vi "Data from tests for IGOR.vi"() -> ()   [LabVIEW 2020]
panel:
  out "G4T vs t Vacuum":cluster{dbl[], dbl[]}(graph)
  out "G4T vs t":T1(graph)
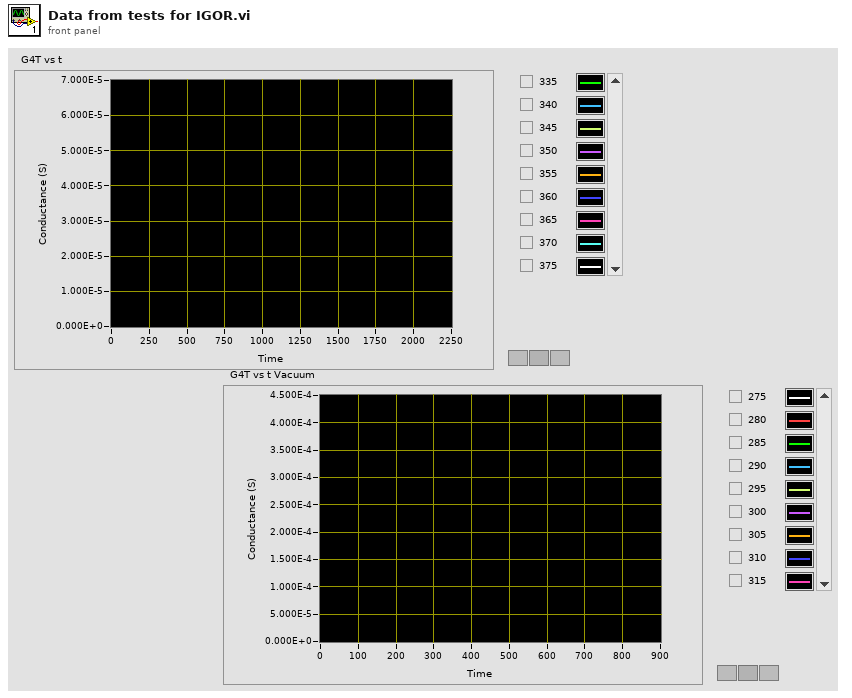
[diagram p1: front panel]
types:
  T1 = cluster{"Data":dbl[], "Best Exponential Fit":dbl[]}[]
  T2 = cluster{"Data":dbl[], "Best Exponential Fit":dbl[]}
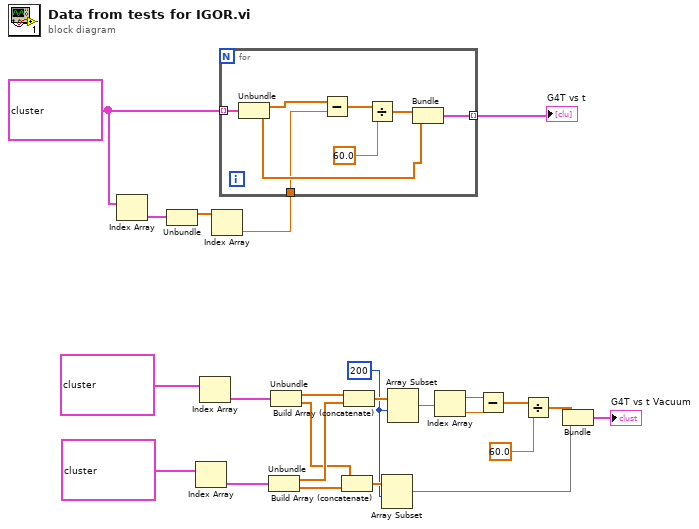
[diagram p0: block diagram]
diagram:
  w1 = 200 ("index")
  w20 = T1 [{"Data"=array[1593 elements], "Best Exponential Fit"=array[1593 elements]}, {"Data"=array[1565 elements], "Best Exponential Fit"=array[1565 elements]}, {"Data"=array[1566 elements], "Best Exponential Fit"=array[1566 elements]}, {"Data"=array[1569 elements], "Best Exponential Fit"=array[1569 elements]}, {"Data"=array[1568 elements], "Best Exponential Fit"=array[1568 elements]}, {"Data"=array[1575 elements], "Best Exponential Fit"=array[1575 elements]}, {"Data"=array[1591 elements], "Best Exponential Fit"=array[1591 elements]}, {"Data"=array[1580 elements], "Best Exponential Fit"=array[1580 elements]}, {"Data"=array[1576 elements], "Best Exponential Fit"=array[1576 elements]}, {"Data"=array[1575 elements], "Best Exponential Fit"=array[1575 elements]}, {"Data"=array[1582 elements], "Best Exponential Fit"=array[1582 elements]}, {"Data"=array[1579 elements], "Best Exponential Fit"=array[1579 elements]}, {"Data"=array[1575 elements], "Best Exponential Fit"=array[1575 elements]}, {"Data"=array[1568 elements], "Best Exponential Fit"=array[1568 elements]}, {"Data"=array[1565 elements], "Best Exponential Fit"=array[1565 elements]}, {"Data"=array[1582 elements], "Best Exponential Fit"=array[1582 elements]}, {"Data"=array[1587 elements], "Best Exponential Fit"=array[1587 elements]}, {"Data"=array[1576 elements], "Best Exponential Fit"=array[1576 elements]}, {"Data"=array[1570 elements], "Best Exponential Fit"=array[1570 elements]}, {"Data"=array[1571 elements], "Best Exponential Fit"=array[1571 elements]}, {"Data"=array[1570 elements], "Best Exponential Fit"=array[1570 elements]}, {"Data"=array[1567 elements], "Best Exponential Fit"=array[1567 elements]}, {"Data"=array[1568 elements], "Best Exponential Fit"=array[1568 elements]}, {"Data"=array[1582 elements], "Best Exponential Fit"=array[1582 elements]}, {"Data"=array[1574 elements], "Best Exponential Fit"=array[1574 elements]}, {"Data"=array[1578 elements], "Best Exponential Fit"=array[1578 elements]}] ("G4T vs t")
  n1 = Index Array(array=w20) -> (element=w21:T2)  [unwired: 1 in]
  n2 = Unbundle(w21) -> ("Data"=w22:dbl[])  [unwired: 1 out]
  n3 = Index Array(array=T1 [{"Data"=array[4227 elements], "Best Exponential Fit"=array[4227 elements]}, {"Data"=array[4227 elements], "Best Exponential Fit"=array[4227 elements]}, {"Data"=array[4227 elements], "Best Exponential Fit"=array[4227 elements]}] ("G vs t vacuum")) -> (element=w11:T2)  [unwired: 1 in]
  n4 = Index Array(array=T1 [{"Data"=array[3134 elements], "Best Exponential Fit"=array[3134 elements]}, {"Data"=array[3134 elements], "Best Exponential Fit"=array[3134 elements]}, {"Data"=array[3134 elements], "Best Exponential Fit"=array[3134 elements]}] ("G vs t heating")) -> (element=w12:T2)  [unwired: 1 in]
  n5 = Index Array(array=w22) -> (element=w19:dbl)  [unwired: 1 in]
  n6 = for {
    tunnel: w20 -> [w31] mode=indexing
    tunnel: [w26] -> w23 mode=indexing
    tunnel: w19 -> [w24]
    n7 = Unbundle(w31) -> ("Data"=w25:dbl[], "Best Exponential Fit"=w27:dbl[])
    n8 = Subtract(x=w25, y=w24) -> (x-y=w30:dbl[])
    n9 = Divide(x=w30, y=60.0) -> (x/y=w28:dbl[])
    n10 = Bundle(w28, "Best Exponential Fit"=w27) -> (w26:cluster{dbl[], "Best Exponential Fit":dbl[]})  [unwired: 1 in]
  }
  "G4T vs t" <- w23
  n11 = Unbundle(w11) -> ("Data"=w16:dbl[], "Best Exponential Fit"=w14:dbl[])
  n12 = Unbundle(w12) -> ("Data"=w15:dbl[], "Best Exponential Fit"=w13:dbl[])
  n13 = Build Array (concatenate)(w13, w14) -> (w5:dbl[])
  n14 = Build Array (concatenate)(w15, w16) -> (w2:dbl[])
  n15 = Array Subset(array=w5, index=w1) -> (w4:dbl[])  [unwired: 1 in]
  n16 = Array Subset(array=w2, index=w1) -> (w3:dbl[])  [unwired: 1 in]
  n17 = Index Array(array=w3) -> (element=w8:dbl)  [unwired: 1 in]
  n18 = Subtract(x=w3, y=w8) -> (x-y=w10:dbl[])
  n19 = Divide(x=w10, y=60.0) -> (x/y=w7:dbl[])
  n20 = Bundle(w7, w4) -> (→"G4T vs t Vacuum":cluster{dbl[], dbl[]})  [unwired: 1 in]
